vi "Set Panel State.vi"(10 "Front Panel Window:State":T1(ring), 11 "Set Panel State in":refnum<class "Set Panel State.lvclass">) -> (3 "Set Panel State out":refnum<class "Set Panel State.lvclass">)   [LabVIEW 2021, in "Set Panel State Msg Strategy.lvlib" / "Set Panel State.lvclass"]
uses:
  Set Panel State.lvclass
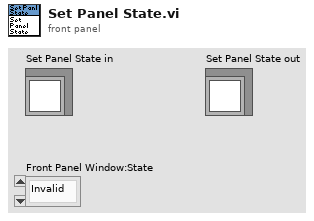
[diagram p1: front panel]
types:
  T1 = enum32{"Invalid", "Standard", "Closed", "Hidden", "Minimized", "Maximized"}
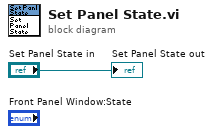
[diagram p0: block diagram]
diagram:
  "Set Panel State out" <- "Set Panel State in"
